vi "data解析.vi"(10 "data_in":u32[](array[numeric]), 11 "格式字符串":string) -> (3 "输出字符串":string)   [LabVIEW 2016]
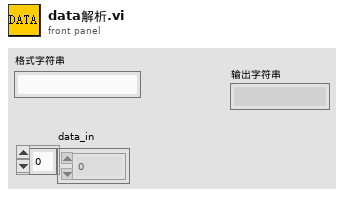
[diagram p1: front panel]
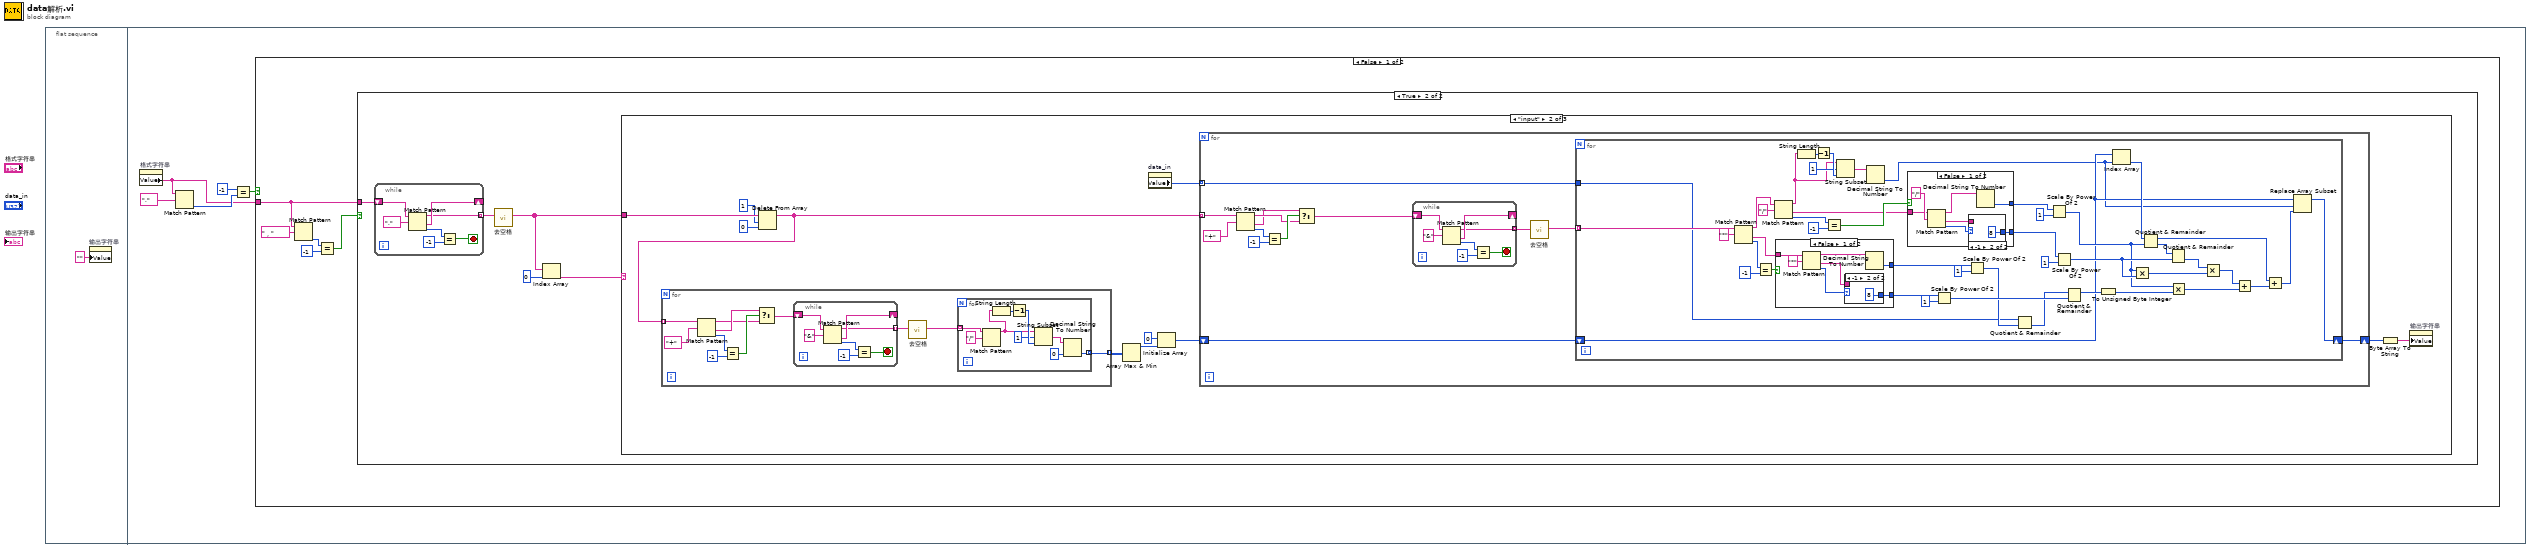
[diagram p0: block diagram]
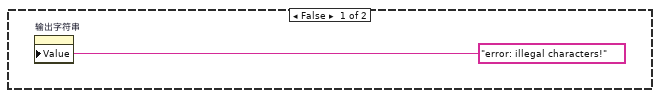
[diagram p2: hidden frame]
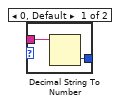
[diagram p4: hidden frame]
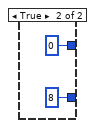
[diagram p5: hidden frame]
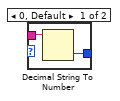
[diagram p6: hidden frame]
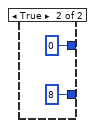
[diagram p7: hidden frame]
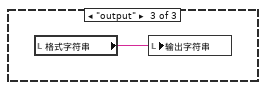
[diagram p8: hidden frame]
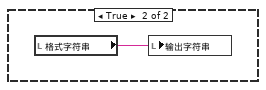
[diagram p9: hidden frame]
diagram:
  n1 = flat-sequence {
    frame #0 {
      n2 = property on="输出字符串" class="Str"("Value"="" ("输出字符串")) -> ()  [unwired: 2 in, 2 out]
    }
    frame #1 {
      n3 = property on="格式字符串" class="Str"() -> ("Value"=w2:string)  [unwired: 2 in, 2 out]
      n4 = Match Pattern(string=w2, regular expression=",") -> (offset past match=w5:i32)  [unwired: 1 in, 3 out]
      n5 = Equal?(x=-1, y=w5) -> (x = y?=w6:bool)
      n6 = case shown="False" w6 {
        tunnel: w2 -> [w11 _]
        frame False {
          n7 = Match Pattern(string=w11, regular expression="，") -> (offset past match=w9:i32)  [unwired: 1 in, 3 out]
          n8 = Equal?(x=w9, y=-1) -> (x = y?=w7:bool)
          n9 = case shown="True" w7 {
            tunnel: w11 -> [_ w17]
            frame False {
              n10 = property on="输出字符串" class="Str"("Value"="error: illegal characters!" ("输出字符串")) -> ()  [unwired: 2 in, 2 out]
            }
            frame True {
              n11 = while {
                shift-right: [w151] -> _
                shift-left: w17 -> [w152]
                tunnel: [w150] -> w16 mode=indexing
                stop <- w146 stop-if-true
                n12 = Match Pattern(string=w152, regular expression=",") -> (before substring=w150:string, after substring=w151:string, offset past match=w148:i32)  [unwired: 1 in, 1 out]
                n13 = Equal?(x=w148, y=-1) -> (x = y?=w146:bool)
              }
              n14 = call "去空格.vi"("Array"=w16) -> ("Array out"=w15:string[])  [unwired: 9 in, 1 out]
              n15 = Index Array(array=w15, index=0) -> (element=w13:string)
              n16 = case shown="\"input\"" w13 {
                tunnel: w15 -> [_ w28 _]
                frame "False", Default {
                }
                frame "input" {
                  n17 = Delete From Array(array=w28, length=1, index=0) -> (array with subset deleted=w25:string[])  [unwired: 1 out]
                  n18 = for {
                    tunnel: w25 -> [w34] mode=indexing
                    tunnel: [w33] -> w24 mode=indexing
                    n19 = Match Pattern(string=w34, regular expression="+") -> (before substring=w30:string, after substring=w31:string, offset past match=w37:i32)  [unwired: 1 in, 1 out]
                    n20 = Equal?(x=w37, y=-1) -> (x = y?=w32:bool)
                    n21 = Select(t=w31, s=w32, f=w30) -> (s? t:f=w29:string)
                    n22 = while {
                      shift-right: [w54] -> _
                      shift-left: w29 -> [w55]
                      tunnel: [w53] -> w35 mode=indexing
                      stop <- w49 stop-if-true
                      n23 = Match Pattern(string=w55, regular expression="&") -> (before substring=w53:string, after substring=w54:string, offset past match=w51:i32)  [unwired: 1 in, 1 out]
                      n24 = Equal?(x=w51, y=-1) -> (x = y?=w49:bool)
                    }
                    n25 = call "去空格.vi"("Array"=w35) -> ("Array out"=w39:string[])  [unwired: 9 in, 1 out]
                    n26 = for {
                      tunnel: w39 -> [w47] mode=indexing
                      tunnel: [w40] -> w33 mode=indexing
                      n27 = Match Pattern(string=w47, regular expression="/") -> (before substring=w43:string)  [unwired: 1 in, 3 out]
                      n28 = String Length(string=w43) -> (length=w45:i32)
                      n29 = Decrement(x=w45) -> (x-1=w46:i32)
                      n30 = String Subset(string=w43, offset (0)=1, length (rest)=w46) -> (substring=w42:string)
                      n31 = Decimal String To Number(string=w42, default (0L)=u32 0 ("default (0 I32)")) -> (number=w40:u32)  [unwired: 1 in, 1 out]
                    }
                  }
                  n32 = Array Max & Min(array=w24) -> (max value=w22:u32)  [unwired: 3 out]
                  n33 = property on="data_in" class="Arr (strict)"() -> ("Value"=w18:u32[])  [unwired: 2 in, 2 out]
                  n34 = Initialize Array(u8 0 ("element"), w22) -> (w21:u8[])
                  n35 = for {
                    tunnel: w25 -> [w64] mode=indexing
                    shift-right: [w61] -> w20
                    shift-left: w21 -> [w62]
                    tunnel: w18 -> [w56] mode=indexing
                    n36 = Match Pattern(string=w64, regular expression="+") -> (before substring=w58:string, after substring=w57:string, offset past match=w66:i32)  [unwired: 1 in, 1 out]
                    n37 = Equal?(x=w66, y=-1) -> (x = y?=w60:bool)
                    n38 = Select(t=w57, s=w60, f=w58) -> (s? t:f=w59:string)
                    n39 = while {
                      shift-right: [w143] -> _
                      shift-left: w59 -> [w144]
                      tunnel: [w142] -> w68 mode=indexing
                      stop <- w138 stop-if-true
                      n40 = Match Pattern(string=w144, regular expression="&") -> (before substring=w142:string, after substring=w143:string, offset past match=w140:i32)  [unwired: 1 in, 1 out]
                      n41 = Equal?(x=w140, y=-1) -> (x = y?=w138:bool)
                    }
                    n42 = call "去空格.vi"("Array"=w68) -> ("Array out"=w63:string[])  [unwired: 9 in, 1 out]
                    n43 = for {
                      tunnel: w63 -> [w106] mode=indexing
                      tunnel: w56 -> [w101]
                      shift-right: [w72] -> w61
                      shift-left: w62 -> [w75]
                      n44 = Match Pattern(string=w106, regular expression="*") -> (before substring=w110:string, after substring=w112:string, offset past match=w70:i32)  [unwired: 1 in, 1 out]
                      n45 = Equal?(x=w70, y=-1) -> (x = y?=w71:bool)
                      n46 = Match Pattern(string=w110, regular expression="/") -> (before substring=w94:string, after substring=w93:string, offset past match=w108:i32)  [unwired: 1 in, 1 out]
                      n47 = case shown="False" w71 {
                        tunnel: w112 -> [w119 _]
                        tunnel: [w116 0] -> w104
                        tunnel: [w115 8] -> w88
                        frame False {
                          n48 = Match Pattern(string=w119, regular expression="*") -> (before substring=w118:string, after substring=w117:string, offset past match=w114:i32)  [unwired: 1 in, 1 out]
                          n49 = case shown="-1" w114 {
                            tunnel: w117 -> [w122 _]
                            tunnel: [w121 8] -> w115
                            frame 0, Default {
                              n50 = Decimal String To Number(string=w122) -> (number=w121:i32)  [unwired: 2 in, 1 out]
                            }
                            frame -1 {
                            }
                          }
                          n51 = Decimal String To Number(string=w118) -> (number=w116:i32)  [unwired: 2 in, 1 out]
                        }
                        frame True {
                        }
                      }
                      n52 = String Length(string=w94) -> (length=w96:i32)
                      n53 = Decrement(x=w96) -> (x-1=w97:i32)
                      n54 = Equal?(x=w108, y=-1) -> (x = y?=w99:bool)
                      n55 = String Subset(string=w94, offset (0)=1, length (rest)=w97) -> (substring=w98:string)
                      n56 = Decimal String To Number(string=w98) -> (number=w74:i32)  [unwired: 2 in, 1 out]
                      n57 = case shown="False" w99 {
                        tunnel: w93 -> [w131 _]
                        tunnel: [w128 0] -> w87
                        tunnel: [w127 8] -> w86
                        frame False {
                          n58 = Match Pattern(string=w131, regular expression="/") -> (before substring=w129:string, after substring=w130:string, offset past match=w126:i32)  [unwired: 1 in, 1 out]
                          n59 = case shown="-1" w126 {
                            tunnel: w130 -> [w134 _]
                            tunnel: [w133 8] -> w127
                            frame 0, Default {
                              n60 = Decimal String To Number(string=w134) -> (number=w133:i32)  [unwired: 2 in, 1 out]
                            }
                            frame -1 {
                            }
                          }
                          n61 = Decimal String To Number(string=w129) -> (number=w128:i32)  [unwired: 2 in, 1 out]
                        }
                        frame True {
                        }
                      }
                      n62 = Scale By Power Of 2(n=w88, x=u32 1) -> (x*2^n=w103:u32)
                      n63 = Scale By Power Of 2(n=w104, x=u32 1) -> (x*2^n=w102:u32)
                      n64 = Quotient & Remainder(x=w101, y=w102) -> (floor(x/y)=w100:u32)  [unwired: 1 out]
                      n65 = Scale By Power Of 2(n=w87, x=u8 1) -> (x*2^n=w82:u8)
                      n66 = Scale By Power Of 2(n=w86, x=u8 1) -> (x*2^n=w85:u8)
                      n67 = Quotient & Remainder(x=w100, y=w103) -> (x-y*floor(x/y)=w81:u32)  [unwired: 1 out]
                      n68 = To Unsigned Byte Integer(number=w81) -> (unsigned 8bit integer=w80:u8)
                      n69 = Index Array(array=w75, index=w74) -> (element=w90:u8)
                      n70 = Multiply(x=w82, y=w85) -> (x*y=w83:u8)
                      n71 = Quotient & Remainder(x=w90, y=w82) -> (x-y*floor(x/y)=w76:u8, floor(x/y)=w89:u8)
                      n72 = Quotient & Remainder(x=w89, y=w85) -> (floor(x/y)=w84:u8)  [unwired: 1 out]
                      n73 = Multiply(x=w82, y=w80) -> (x*y=w78:u8)
                      n74 = Multiply(x=w84, y=w83) -> (x*y=w79:u8)
                      n75 = Add(x=w79, y=w78) -> (x+y=w77:u8)
                      n76 = Add(x=w76, y=w77) -> (x+y=w73:u8)
                      n77 = Replace Array Subset(array=w75, new element=w73, index=w74) -> (w72:u8[])
                    }
                  }
                  n78 = Byte Array To String(unsigned byte array=w20) -> (string=w19:string)
                  n79 = property on="输出字符串" class="Str"("Value"=w19) -> ()  [unwired: 2 in, 2 out]
                }
                frame "output" {
                  n80 = local read "格式字符串"() -> (w145:string)
                  n81 = local write "输出字符串"(w145) -> ()
                }
              }
            }
          }
        }
        frame True {
          n82 = local read "格式字符串"() -> (w153:string)
          n83 = local write "输出字符串"(w153) -> ()
        }
      }
    }
  }
